vi "set filter (custom).vi"(8 "error in (no error)":errorcluster, 11 "abstract-tree in":refnum<class "abstract-tree.lvclass">) -> (0 "error out":errorcluster, 3 "abstract-tree out":refnum<class "abstract-tree.lvclass">)   [LabVIEW 2017, in "vs-tree-utility.lvlib" / "abstract-tree.lvclass"]
uses:
  abstract-tree.lvclass
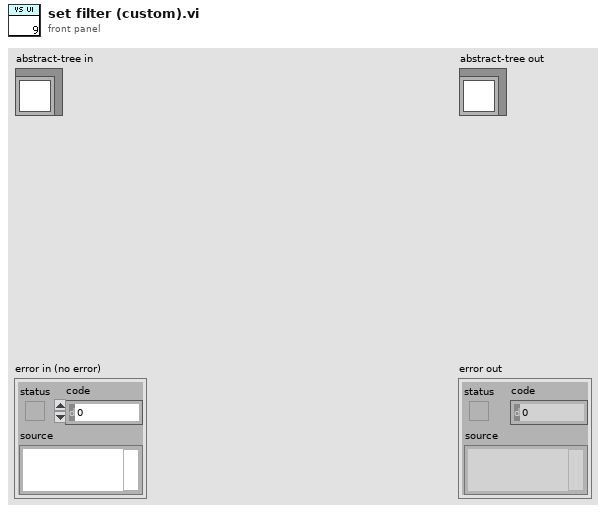
[diagram p1: front panel]
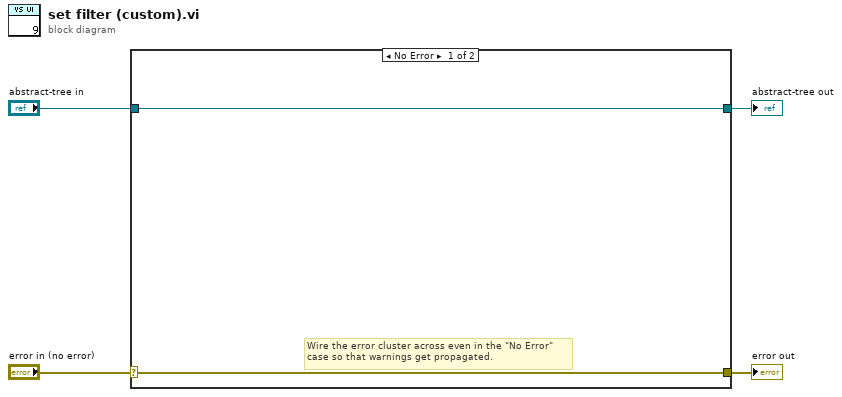
[diagram p0: block diagram]
diagram:
  n1 = case shown="No Error" "error in (no error)" {
    selector: "error in (no error)" -> [w5 w8]
    tunnel: [w5 w8] -> w3
    tunnel: [w6 w7] -> w1
    tunnel: "abstract-tree in" -> [w6 w7]
    frame No Error {
      # "Wire the error cluster across even in the \"No Error\"\ncase so that warnings get propagated."
    }
    frame Error {
    }
  }
  "error out" <- w3
  "abstract-tree out" <- w1
